vi "Periodic.Tasks.vi"(8 "error in":errorcluster) -> ()   [LabVIEW 2015]
doc: "This VI runs in parallel to other tasks. It can contain as many user-defined periodic loops as you need. These can carry out PID or other sorts of timed response."
uses:
  <vilib>/Rock Robotics/Network Tables/NT Write Number.vi
  <vilib>/Rock Robotics/WPI/Utilities/WPI_GetSetVariantRefNum.vi
  Robot Global Data.vi
  <vilib>/addons/control/pid/pid.llb/PID (DBL).vi
  <vilib>/Rock Robotics/WPI/RobotDrive/WPI_RobotDriveArcadeDrive_Standard(NoSaturation).vi
  navX Library v2/navX Library v2.lvlib
  <vilib>/addons/control/pid/NI_PID_pid.lvlib
panel:
  in  "PID gains":T1={"proportional gain (Kc)"=1.0, "integral time (Ti, min)"=0.0, "derivative time (Td, min)"=0.0} {"derivative time (Td, min)" format="%.3f"; "integral time (Ti, min)" format="%.3f"; "proportional gain (Kc)" format="%.3f"}
  in  "Min":dbl=0.5
  in  "Max":dbl=0.75
  in  "Reset Gyro":bool
  out "gyro":dbl
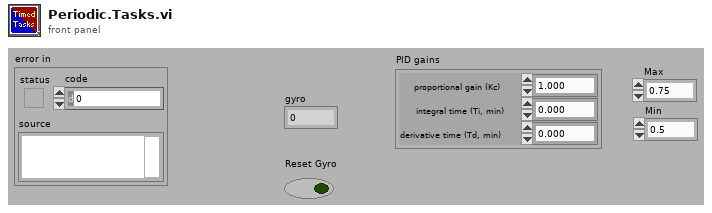
[diagram p1: front panel]
types:
  T1 = cluster{"proportional gain (Kc)":dbl, "integral time (Ti, min)":dbl, "derivative time (Td, min)":dbl}
  T2 = typedef "WPI_EncoderDevRef.ctl" = cluster{"DevStatus":errorcluster, "EncoderIndex":T3, "CounterIndex":T4, "DistancePerCount":dbl, "Decoding Type":T5}
  T3 = typedef "FPGA_EncoderIdx.ctl" = enum8{"Enc 0", "Enc 1", "Enc 2", "Enc 3", "Enc 4", "Enc 5", "Enc 6", "Enc 7", "Invalid"}
  T4 = typedef "FPGA_CounterCtrSystemIndex.ctl" = enum8{"Ctr 0", "Ctr 1", "Ctr 2", "Ctr 3", "Ctr 4", "Ctr 5", "Ctr 6", "Ctr 7", "Invalid"}
  T5 = typedef "WPI_EncoderType.ctl" = enum16{"1x", "2x", "4x"}
  T6 = typedef "navX Library v2.lvlib/Z900_navX_DeviceTypeDef.ctl" = cluster{"Interface":cluster{"Protocol":T7, "Update Rate (4Hz-60Hz)":u8, "navX Open TypeDef":variant}, "Notify Packet":refnum<notifier>, "Loop VI Refnum":refnum<vi>, "Ready to Close Occurrence Refnum":refnum<k4>}
  T7 = typedef "navX Library v2.lvlib/Z900_navX_ProtocolTypeDef.ctl" = enum16{"SERIAL", "I2C", "SPI"}
  T8 = cluster{"Yaw":dbl, "Roll":dbl, "Pitch":dbl, "Heading":dbl, "Fused Heading":dbl}
  T9 = typedef "WPI_AnalogChannelDevRef.ctl" = cluster{"DevStatus":errorcluster, "Analog Channel":T10}
  T10 = typedef "FPGA_AIChannel.ctl" = enum8{"AI 0", "AI 1", "AI 2", "AI 3", "AI MXP 0", "AI MXP 1", "AI MXP 2", "AI MXP 3", "Invalid"}
  T11 = typedef "WPI_MotorControlDeviceRef.ctl" = cluster{"DeviceStatus":errorcluster, "Type":T12, "PWM":cluster{"PWM Channel":T13, "DeadBand":T14}, "CAN":cluster{"Device Number":u8, "Control Mode":T15, "Semaphore":T16, "Max Vout":dbl, "TalonSRX Control Mode":T17}, "Invert":bool}
  T12 = typedef "WPI_MotorControlType.ctl" = enum16{"PWM", "CAN", "CANTalonSRX"}
  T13 = typedef "FPGA_DIOPWMChannel.ctl" = enum8{"PWM 0", "PWM 1", "PWM 2", "PWM 3", "PWM 4", "PWM 5", "PWM 6", "PWM 7", "PWM 8", "PWM 9", "PWM MXP 0", "PWM MXP 1", "PWM MXP 2", "PWM MXP 3", "PWM MXP 4", "PWM MXP 5", "PWM MXP 6", "PWM MXP 7", "PWM MXP 8", "PWM MXP 9", "Invalid"}
  T14 = typedef "WPI_PWMDeadband.ctl" = cluster{"Name":string, "maxPositivePwm":i32, "minPositivePwm":i32, "centerPwm":i32, "maxNegativePwm":i32, "minNegativePwm":i32, "angularRange":u16}
  T15 = typedef "WPI_CANJaguar_ControlMode.ctl" = enum8{"Percent VBus", "Current", "Speed", "Position", "Voltage"}
  T16 = typedef "Semaphore RefNum" = refnum<k1>
  T17 = typedef "WPI_CANTalonSRX_APIControlMode.ctl" = enum8{"Percent VBus", "Speed", "Position", "Slave", "Unchanged / Invalid", "Voltage Compensation", "Current", "Motion Profile"}
  T18 = typedef "WPI_ServoDeviceRef.ctl" = cluster{"DeviceStatus":errorcluster, "PWM Channel":T13, "DeadBand":T14}
  T19 = typedef "WPI_RobotDriveDevRef.ctl" = cluster{"DevStatus":errorcluster, "Motors[]":T11[], "Square Inputs":bool, "Max Output":dbl}
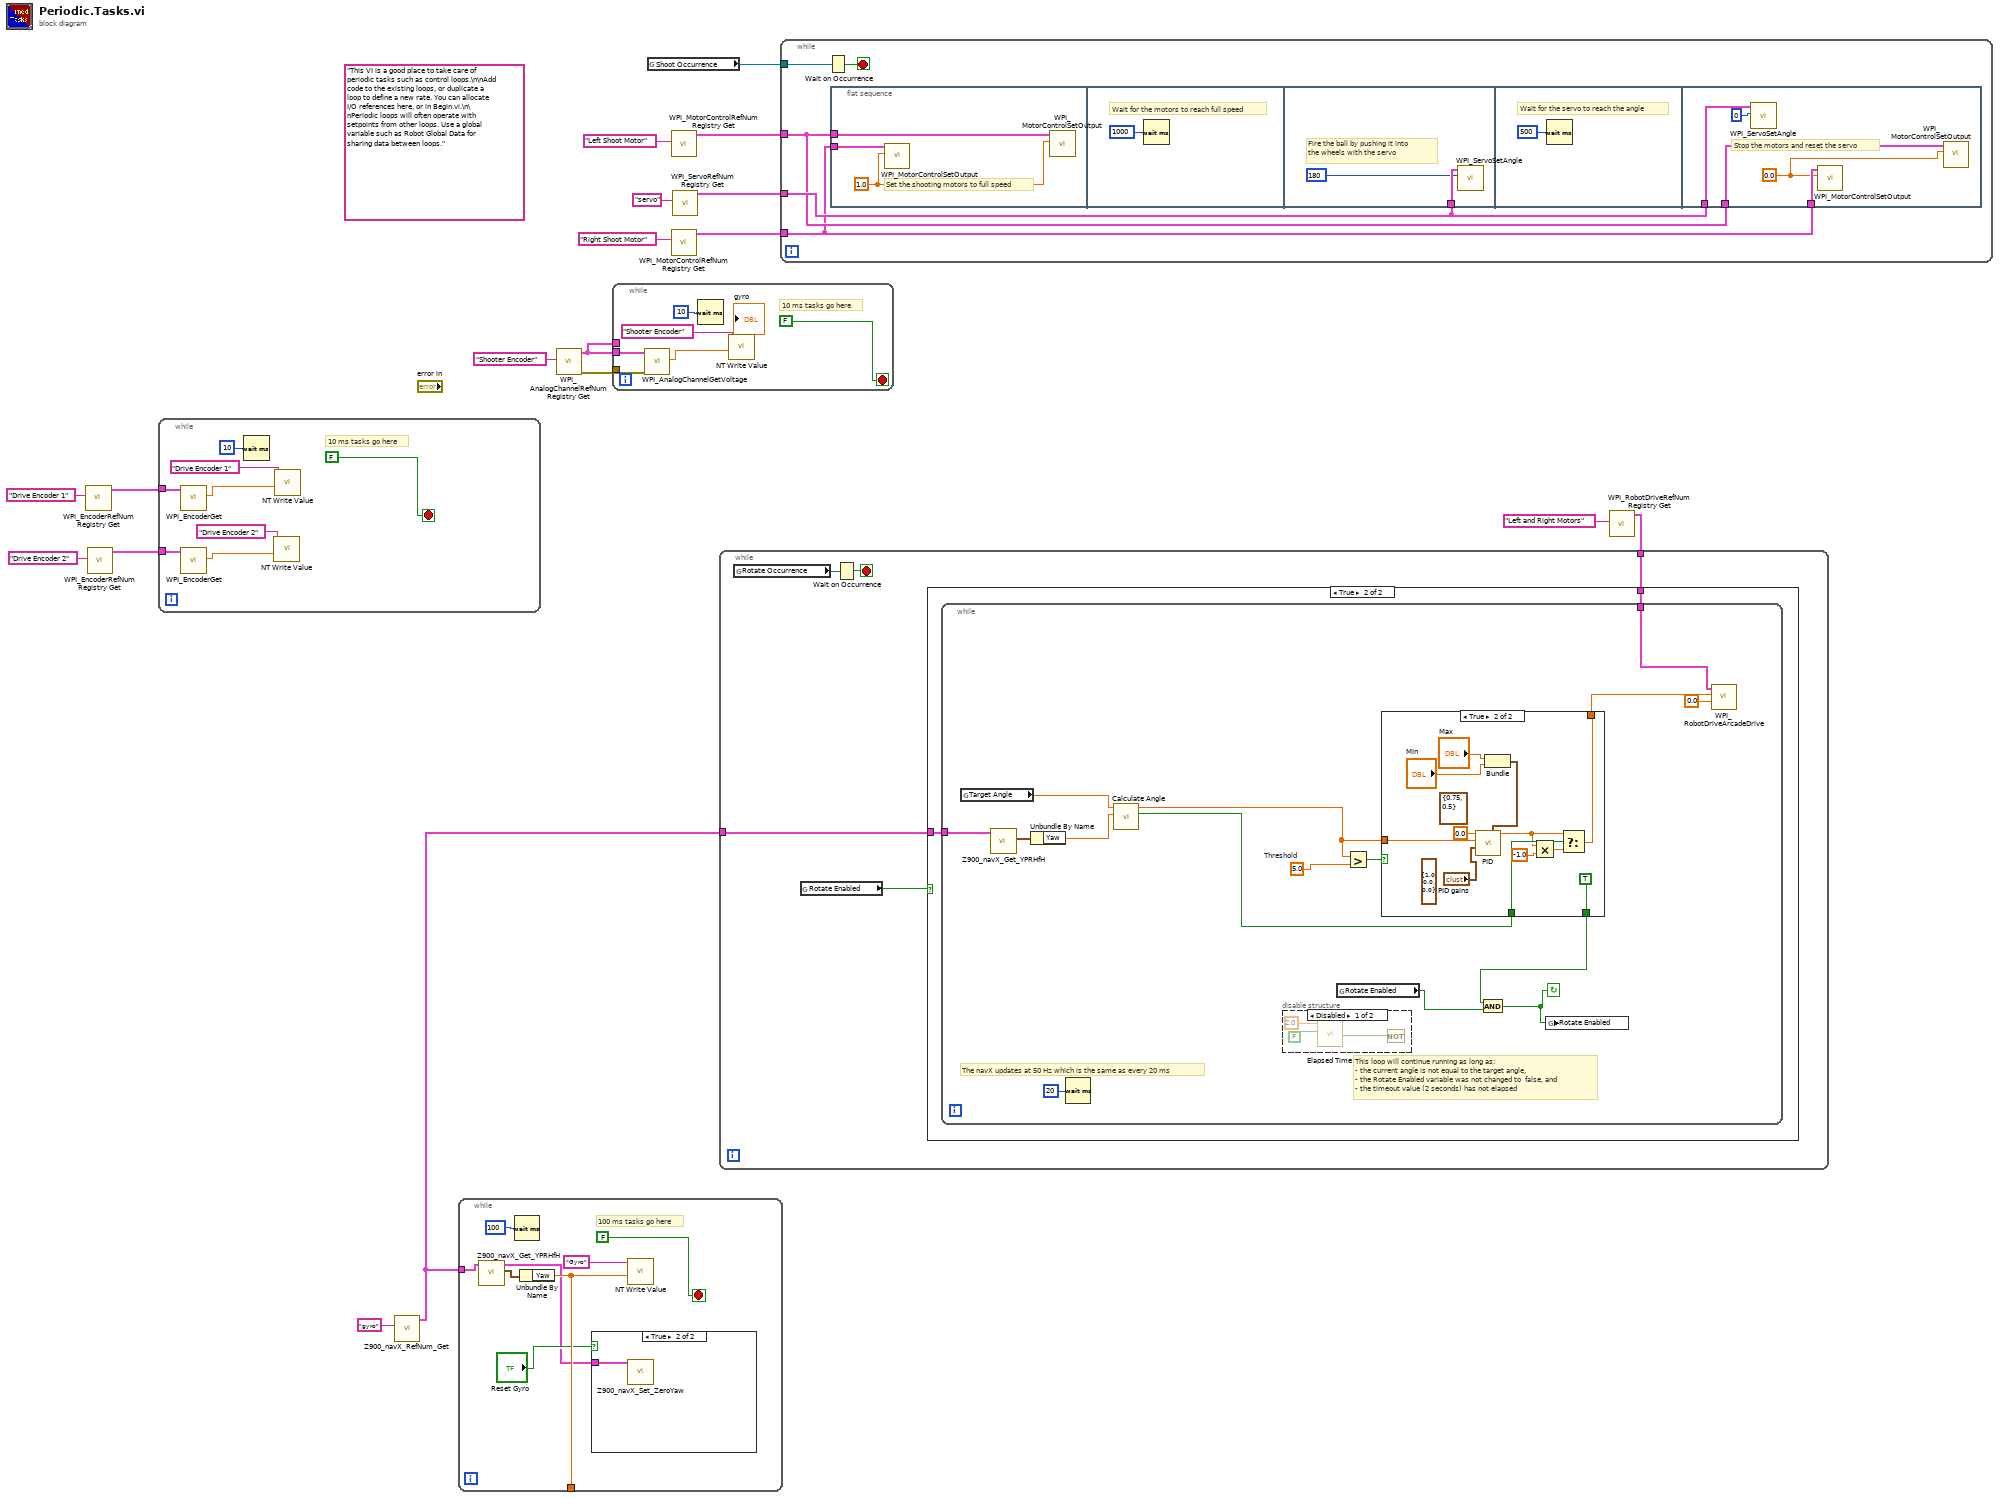
[diagram p0: block diagram]
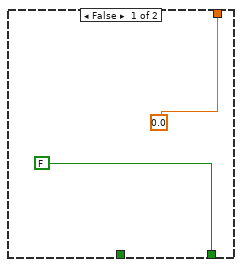
[diagram p4: hidden frame]
diagram:
  (unwired) "This VI is a good place to take care of periodic tasks such as control loops.\n\nAdd code to the existing loops, or duplicate a loop to define a new rate. You can allocate I/O references here, or in Begin.vi.\n\nPeriodic loops will often operate with setpoints from other loops. Use a global variable such as Robot Global Data for sharing data between loops."
  n1 = call <vilib>:"WPI_EncoderRefNum Registry Get.vi"("refnum name"="Drive Encoder 1") -> ("EncoderDevRef"=w7:T2)  [unwired: 9 in, 1 out]
  n2 = call <vilib>:"WPI_EncoderRefNum Registry Get.vi"("refnum name"="Drive Encoder 2") -> ("EncoderDevRef"=w6:T2)  [unwired: 9 in, 1 out]
  n3 = while {
    tunnel: w7 -> [w23]
    tunnel: w6 -> [w22]
    stop <- FALSE stop-if-true
    # "10 ms tasks go here"
    n4 = call <vilib>:"WPI_EncoderGet.vi"("EncoderDevRef"=w23) -> ("Distance"=w19:dbl)  [unwired: 5 in, 5 out]
    n5 = call <vilib>:"WPI_EncoderGet.vi"("EncoderDevRef"=w22) -> ("Distance"=w20:dbl)  [unwired: 5 in, 5 out]
    n6 = Wait (ms)(milliseconds to wait=u32 10) -> ()  [unwired: 1 out]
    n7 = call-poly <vilib>:"NT Write Value.vi"("Numeric"=w20, "Name"="Drive Encoder 2") -> ()  [unwired: 9 in, 1 out]
    n8 = call-poly <vilib>:"NT Write Value.vi"("Numeric"=w19, "Name"="Drive Encoder 1") -> ()  [unwired: 9 in, 1 out]
  }
  n9 = call "Z900_navX_RefNum_Get.vi"("refnum name"="gyro") -> ("navX Device"=w3:T6)  [unwired: 9 in, 1 out]
  n10 = while {
    tunnel: w3 -> [w30]
    tunnel: [w29] -> _
    stop <- FALSE stop-if-true
    # "100 ms tasks go here"
    n11 = call "Z900_navX_Get_YPRHfH.vi"("navX Device"=w30) -> ("YRPHfH"=w31:T8, "navX Device"=w27:T6)  [unwired: 7 in, 2 out]
    n12 = Wait (ms)(milliseconds to wait=u32 100) -> ()  [unwired: 1 out]
    n13 = Unbundle By Name(w31) -> ("Yaw"=w29:dbl)
    n14 = case shown="True" "Reset Gyro" {
      tunnel: w27 -> [_ w35]
      frame False {
      }
      frame True {
        n15 = call "Z900_navX_Set_ZeroYaw.vi"("navX Device"=w35) -> ()  [unwired: 9 in, 2 out]
      }
    }
    n16 = call-poly <vilib>:"NT Write Value.vi"("Numeric"=w29, "Name"="Gyro") -> ()  [unwired: 9 in, 1 out]
  }
  n17 = call <vilib>:"WPI_AnalogChannelRefNum Registry Get.vi"("refnum name"="Shooter Encoder") -> ("error out"=w11:errorcluster, "AIDeviceRef"=w12:T9)  [unwired: 9 in]
  n18 = while {
    tunnel: w12 -> [_]
    tunnel: w12 -> [w38]
    tunnel: w11 -> [w36]
    stop <- FALSE stop-if-true
    # "10 ms tasks go here"
    n19 = call <vilib>:"WPI_AnalogChannelGetVoltage.vi"("error in (no error)"=w36, "AIDeviceRef"=w38) -> ("Voltage"=w37:dbl)  [unwired: 7 in, 2 out]
    n20 = Wait (ms)(milliseconds to wait=u32 10) -> ()  [unwired: 1 out]
    n21 = call-poly <vilib>:"NT Write Value.vi"("Numeric"=w37, "Name"="Shooter Encoder") -> ()  [unwired: 9 in, 1 out]
  }
  n22 = global read "Robot Global Data.vi" "Shoot Occurrence"() -> (w16:refnum<k4>)
  n23 = call <vilib>:"WPI_MotorControlRefNum Registry Get.vi"("refnum name"="Left Shoot Motor") -> ("MotorControlDevRef"=w8:T11)  [unwired: 9 in, 1 out]
  n24 = call <vilib>:"WPI_MotorControlRefNum Registry Get.vi"("refnum name"="Right Shoot Motor") -> ("MotorControlDevRef"=w10:T11)  [unwired: 9 in, 1 out]
  n25 = call <vilib>:"WPI_ServoRefNum Registry Get.vi"("refnum name"="servo") -> ("ServoDeviceRef"=w9:T18)  [unwired: 9 in, 1 out]
  n26 = while {
    tunnel: w10 -> [w42]
    tunnel: w8 -> [w43]
    tunnel: w16 -> [w45]
    tunnel: w9 -> [w44]
    stop <- w46 stop-if-true
    n27 = Wait on Occurrence(2:w45) -> (0:w46:bool)  [unwired: 2 in]
    n28 = flat-sequence {
      tunnel: w42 -> [w48]
      tunnel: w43 -> [w47]
      tunnel: w44 -> [w52]
      tunnel: w44 -> [w57]
      tunnel: w43 -> [w56]
      tunnel: w42 -> [w55]
      frame #0 {
        w49 = 1.0 ("Output")
        # "Set the shooting motors to full speed"
        n29 = call <vilib>:"WPI_MotorControlSetOutput.vi"("Output"=w49, "MotorControlDevRef"=w48) -> ()  [unwired: 7 in, 3 out]
        n30 = call <vilib>:"WPI_MotorControlSetOutput.vi"("Output"=w49, "MotorControlDevRef"=w47) -> ()  [unwired: 7 in, 3 out]
      }
      frame #1 {
        # "Wait for the motors to reach full speed"
        n31 = Wait (ms)(milliseconds to wait=u32 1000) -> ()  [unwired: 1 out]
      }
      frame #2 {
        # "Fire the ball by pushing it into the wheels with the servo"
        n32 = call <vilib>:"WPI_ServoSetAngle.vi"("Angle"=180, "ServoDeviceRef"=w52) -> ()  [unwired: 8 in, 2 out]
      }
      frame #3 {
        # "Wait for the servo to reach the angle"
        n33 = Wait (ms)(milliseconds to wait=u32 500) -> ()  [unwired: 1 out]
      }
      frame #4 {
        w54 = 0.0 ("Output")
        # "Stop the motors and reset the servo"
        n34 = call <vilib>:"WPI_ServoSetAngle.vi"("Angle"=0, "ServoDeviceRef"=w57) -> ()  [unwired: 8 in, 2 out]
        n35 = call <vilib>:"WPI_MotorControlSetOutput.vi"("Output"=w54, "MotorControlDevRef"=w55) -> ()  [unwired: 7 in, 3 out]
        n36 = call <vilib>:"WPI_MotorControlSetOutput.vi"("Output"=w54, "MotorControlDevRef"=w56) -> ()  [unwired: 7 in, 3 out]
      }
    }
  }
  n37 = call <vilib>:"WPI_RobotDriveRefNum Registry Get.vi"("refnum name"="Left and Right Motors") -> ("RobotDriveDevRef"=w1:T19)  [unwired: 1 in, 9 out]
  n38 = while {
    tunnel: w3 -> [w60]
    tunnel: w1 -> [w59]
    stop <- w62 stop-if-true
    n39 = global read "Robot Global Data.vi" "Rotate Occurrence"() -> (w63:refnum<k4>)
    n40 = global read "Robot Global Data.vi" "Rotate Enabled"() -> (w61:bool)
    n41 = Wait on Occurrence(2:w63) -> (0:w62:bool)  [unwired: 2 in]
    n42 = case shown="True" w61 {
      tunnel: w60 -> [_ w65]
      tunnel: w59 -> [_ w64]
      frame False {
      }
      frame True {
        n43 = while {
          tunnel: w65 -> [w75]
          tunnel: w64 -> [w68]
          stop <- w70 continue-if-true
          w77 = 5.0  # Threshold
          # "The navX updates at 50 Hz which is the same as every 20 ms"
          # "This loop will continue running as long as:\n- the current angle is not equal to the target angle,\n- the Rotate Enabled variable was not changed to  false, and\n- the timeout value (2 seconds) has not elapsed"
          n44 = global read "Robot Global Data.vi" "Target Angle"() -> (w74:dbl)
          n45 = call "Z900_navX_Get_YPRHfH.vi"("navX Device"=w75) -> ("YRPHfH"=w76:T8)  [unwired: 7 in, 3 out]
          n46 = Unbundle By Name(w76) -> ("Yaw"=w73:dbl)
          n47 = Wait (ms)(milliseconds to wait=u32 20) -> ()  [unwired: 1 out]
          n48 = call "Calculate Angle.vi"("Current Angle"=w73, "Target Angle"=w74) -> ("Clockwise"=w72:bool, "Delta Angle"=w69:dbl)  [unwired: 8 in]
          n49 = disable-structure shown="Disabled" {
            frame Disabled {
              n50 = call "Elapsed Time"("Time Target (s)"=2.0, "Reset"=FALSE) -> ("Time has Elapsed"=w81:bool)  [unwired: 10 in, 7 out]
              n51 = Not(x=w81) -> ()  [unwired: 1 out]
            }
            frame Enabled {
            }
          }
          n52 = global read "Robot Global Data.vi" "Rotate Enabled"() -> (w71:bool)
          n53 = Greater?(x=w69, y=w77) -> (0:w78:bool)
          n54 = case shown="True" w78 {
            tunnel: [0.0 ("Left axis value") w96] -> w67
            tunnel: w72 -> [_ w95]
            tunnel: [FALSE ("Rotate Enabled") TRUE ("Rotate Enabled")] -> w80
            tunnel: w69 -> [_ w91]
            frame False {
            }
            frame True {
              (unwired) T1 {"proportional gain (Kc)"=1.0, "integral time (Ti, min)"=0.0, "derivative time (Td, min)"=0.0} ("PID gains")
              (unwired) cluster{"output high":dbl, "output low":dbl} {"output high"=0.75, "output low"=0.5} ("output range")
              n55 = Bundle("Max"="Max", "Min"="Min") -> (w87:cluster{"Max":dbl, "Min":dbl})  [unwired: 1 in]
              n56 = call-poly <vilib>:"PID.vi"("output range"=w87, "PID gains"="PID gains", "process variable"=w91, "setpoint"=0.0) -> ("output"=w92:dbl)  [unwired: 6 in, 1 out]
              n57 = Multiply(x=w92, y=-1.0) -> (x*y=w94:dbl)
              n58 = Select(t=w92, s=w95, f=w94) -> (s? t:f=w96:dbl)
            }
          }
          n59 = Compound Arithmetic op=AND(w80, w71) -> (w70:bool)
          n60 = global write "Robot Global Data.vi" "Rotate Enabled"(w70) -> ()
          n61 = call-poly <vilib>:"WPI_RobotDriveArcadeDrive.vi"("Y axis value"=0.0, "X axis value"=w67, "RobotDriveDevRef"=w68) -> ()  [unwired: 6 in, 3 out]
        }
      }
    }
  }
